vi "GenericResponse_Parse.vi"(8 "error in (no error)":errorcluster, 11 "Message":T5) -> (0 "error out":errorcluster, 1 "Body":T1, 2 "Header":T3, 3 "GenericResponse":T2)   [LabVIEW 2017]
uses:
  <vilib>/addons/InsightCM/MessageBus/Base/controls/Message.ctl
  <vilib>/addons/InsightCM/MessageBus/Base/controls/MessageHeader.ctl
  <vilib>/addons/InsightCM/MessageBus/Base/controls/KeyValuePair.ctl
  <vilib>/addons/InsightCM/MessageBus/Base/controls/GenericResponse.ctl
  <vilib>/addons/InsightCM/MessageBus/Base/controls/GenericResponseBody.ctl
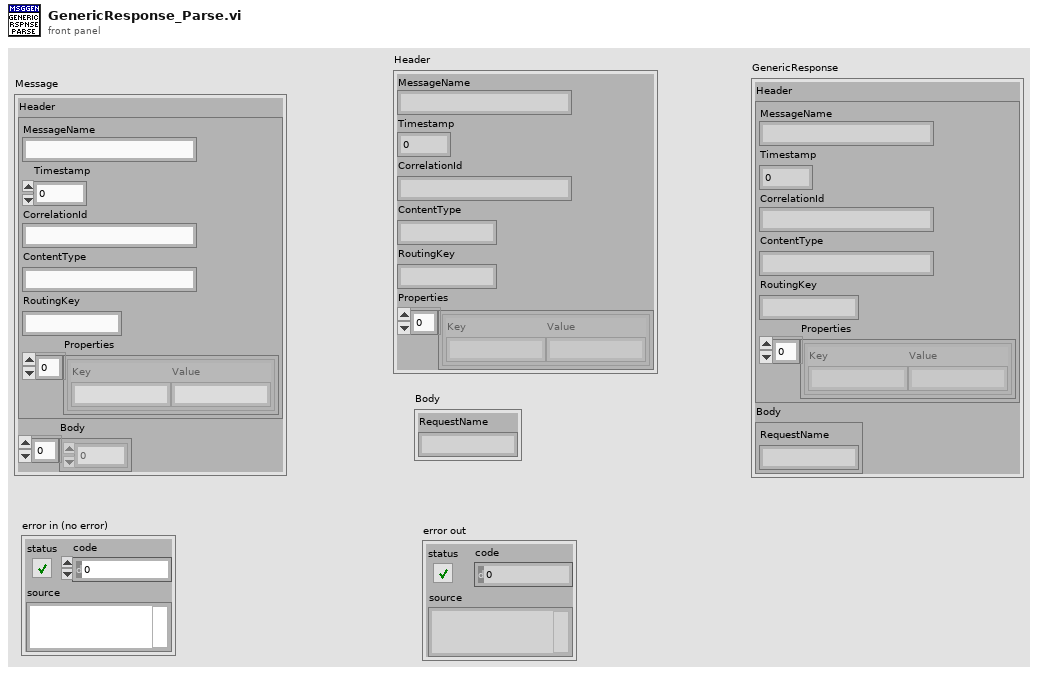
[diagram p1: front panel]
types:
  T1 = typedef "GenericResponseBody.ctl" = cluster{"RequestName":string}
  T2 = typedef "GenericResponse.ctl" = cluster{"Header":T3, "Body":T1}
  T3 = typedef "MessageHeader.ctl" = cluster{"MessageName":string, "Timestamp":i64, "CorrelationId":string, "ContentType":string, "RoutingKey":string, "Properties":T4[]}
  T4 = typedef "KeyValuePair.ctl" = cluster{"Key":string, "Value":string}
  T5 = typedef "Message.ctl" = cluster{"Header":T3, "Body":u8[]}
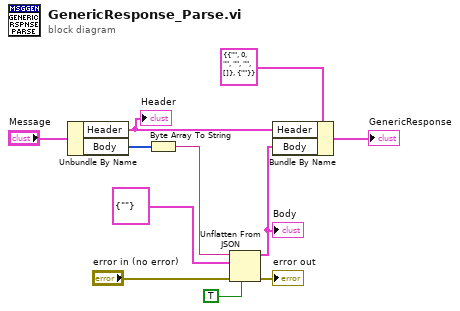
[diagram p0: block diagram]
diagram:
  n1 = Unbundle By Name("Message") -> ("Header"=w9:T3, "Body"=w3:u8[])
  "Header" <- w9
  n2 = Byte Array To String(unsigned byte array=w3) -> (string=w7:string)
  n3 = Unflatten From JSON(JSON string=w7, type and defaults=T1 {"RequestName"=""} ("Body"), default null elements? (F)=TRUE, error in (no error)="error in (no error)") -> (value=w6:T1, error out=→"error out":errorcluster)  [unwired: 3 in]
  "Body" <- w6
  n4 = Bundle By Name(cluster=T2 {"Header"={"MessageName"="", "Timestamp"=0, "CorrelationId"="", "ContentType"="", "RoutingKey"="", "Properties"=[]}, "Body"={"RequestName"=""}} ("GenericResponse"), "Header"=w9, "Body"=w6) -> (→"GenericResponse":T2)
